vi "Write MAP DVR.vi"(8 "error in (no error)":errorcluster, 10 "MAP DVR":refnum<data-value>, 11 "Exe Write Main in":refnum<class "Exe Write PAS Waveforms.lvclass">) -> (0 "error out":errorcluster, 3 "Exe Write Main out":refnum<class "Exe Write PAS Waveforms.lvclass">)   [LabVIEW 2014, in "Controller.lvlib" / "Exe Write PAS Waveforms.lvclass"]
uses:
  Exe Write PAS Waveforms.lvclass
  Exe Write PAS Waveforms.lvclass/Exe Write PAS Waveforms.ctl
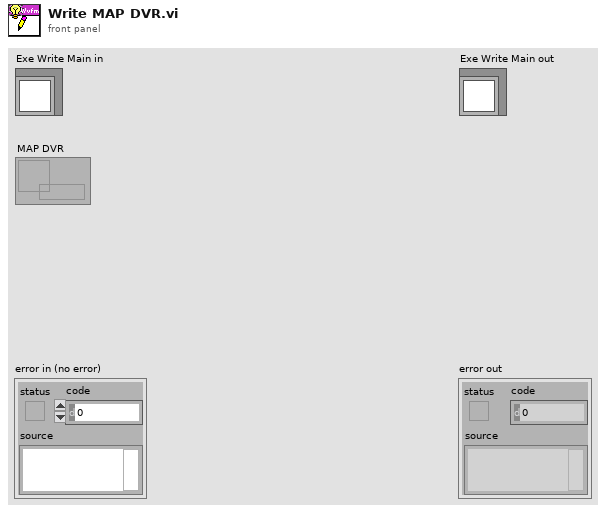
[diagram p1: front panel]
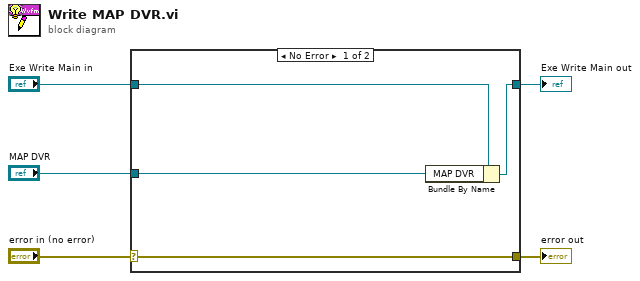
[diagram p0: block diagram]
diagram:
  n1 = case shown="No Error" "error in (no error)" {
    selector: "error in (no error)" -> [w9 w10]
    tunnel: [w9 w10] -> w4
    tunnel: [w7 w11] -> w2
    tunnel: "Exe Write Main in" -> [w8 w11]
    tunnel: "MAP DVR" -> [w6 _]
    frame No Error {
      n2 = Bundle By Name(cluster=w8, "MAP DVR"=w6) -> (w7:refnum<class "Exe Write PAS Waveforms.lvclass">)
    }
    frame Error {
    }
  }
  "error out" <- w4
  "Exe Write Main out" <- w2
